vi "Check Expected Heartbeats.vi"(8 "Error In":errorcluster, 11 "reference in":refnum<class "Network Mangement.lvclass">) -> (0 "Error Out":errorcluster, 3 "reference out":refnum<class "Network Mangement.lvclass">)   [LabVIEW 2024, in "Network Mangement.lvclass"]
uses:
  Network Mangement.lvclass
panel:
  out "Overdue?":bool[](array[boolean])
  out "Node IDs":u8[](array[numeric])
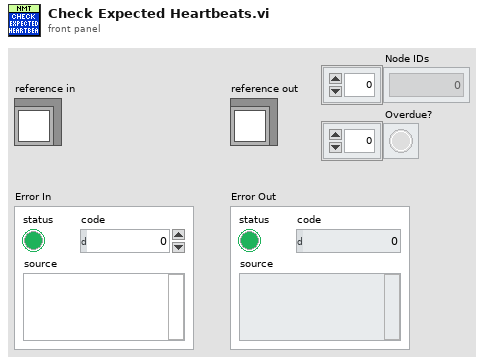
[diagram p1: front panel]
types:
  T1 = typedef "Network Mangement.lvclass/ObjectAttributes.ctl" = cluster{"Nodes":map{u8, u8}, "Heartbeats":map{u8, cluster{"Period":u16, "Timeout":u16, "Last Beat":timestamp}}, "Events":cluster{"Stop Heartbeat Checker":refnum<user-event>, "Heartbeat Timeout":refnum<user-event>, "Heartbeat Checker Error":refnum<user-event>}, "Heartbeat Checker":refnum<vi>}
  T2 = map{u8, cluster{"Period":u16, "Timeout":u16, "Last Beat":timestamp}}
  T3 = cluster{"Period":u16, "Timeout":u16, "Last Beat":timestamp}
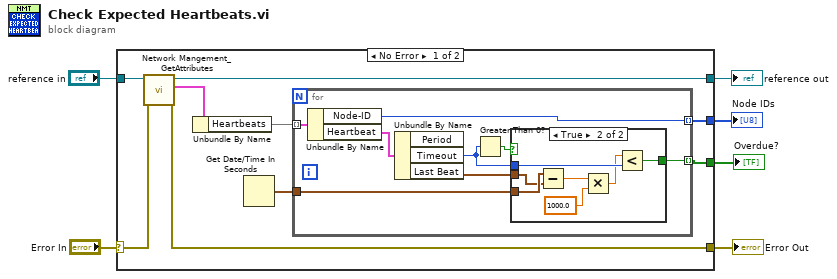
[diagram p0: block diagram]
diagram:
  n1 = case shown="No Error" "Error In" {
    selector: "Error In" -> [w15 w32]
    tunnel: [w13 w32] -> w5
    tunnel: [w11 w31] -> w3
    tunnel: "reference in" -> [w12 w31]
    tunnel: [w8 _] -> w2
    tunnel: [w7 _] -> w1
    frame No Error {
      n2 = call "Network Mangement_GetAttributes.vi"("Error In"=w15, "reference in"=w12) -> ("Error Out"=w13:errorcluster, "Data"=w14:T1, "reference out"=w11:refnum<class "Network Mangement.lvclass">)  [unwired: 6 in, 1 out]
      n3 = Unbundle By Name(w14) -> ("Heartbeats"=w10:T2)
      n4 = Get Date/Time In Seconds() -> (seconds since 1Jan1904=w9:timestamp)
      n5 = for {
        tunnel: w10 -> [w23] mode=indexing
        tunnel: [w20] -> w7 mode=indexing
        tunnel: [w19] -> w8 mode=indexing
        tunnel: w9 -> [w18]
        n6 = Unbundle By Name(w23) -> ("Node-ID"=w19:u8, "Heartbeat"=w22:T3)
        n7 = Unbundle By Name(w22) -> ("Timeout"=w17:u16, "Last Beat"=w21:timestamp)  [unwired: 1 out]
        n8 = Greater Than 0?(x=w17) -> (x > 0?=w16:bool)
        n9 = case shown="True" w16 {
          tunnel: w21 -> [_ w27]
          tunnel: w17 -> [_ w30]
          tunnel: [_ w29] -> w20
          tunnel: w18 -> [_ w28]
          frame False {
          }
          frame True {
            n10 = Subtract(x=w28, y=w27) -> (x-y=w26:dbl)
            n11 = Multiply(x=w26, y=1000.0) -> (x*y=w25:dbl)
            n12 = Less?(x=w25, y=w30) -> (x < y?=w29:bool)
          }
        }
      }
    }
    frame Error {
    }
  }
  "Error Out" <- w5
  "reference out" <- w3
  "Node IDs" <- w2
  "Overdue?" <- w1
